vi "Init_Horizontal_ROI.vi"(8 "error in (no error)":errorcluster, 10 "input cluster":T1={"Mode"=enum."ROI", "Manual LUT"={"Minimum"=0.0, "Maximum"=0.0}, "BCG Values"={"Brightness"=128.0, "Contrast"=45.0, "Gamma"=1.0}, "ImageProcessed"=refnum, "Image "=refnum, "Log?"=FALSE, "Auto?"=FALSE, "ROI"={"Global Rectangle"=[], "Contours"=[]}, "ROI Parameters"={"Count"=0.0, "Size(um)"=0.0}, "Image X"=0, "Image Y"=0, "Horizontal ROI"={"Global Rectangle"=[], "Contours"=[]}, "HROI Pos"=0, "Custom ROI"={"Global Rectangle"=[], "Contours"=[]}, "Intensity Graph"=[]} {"ROI Parameters"."Size(um)" min=0 max=255 step=0.1 format="%.2f"; "ROI Parameters"."Count" min=0 max=255 step=0.1 format="%.2f"}) -> (0 "error out":errorcluster, 2 "output cluster":T1={"Mode"=enum."ROI", "Manual LUT"={"Minimum"=0.0, "Maximum"=0.0}, "BCG Values"={"Brightness"=128.0, "Contrast"=45.0, "Gamma"=1.0}, "ImageProcessed"=refnum, "Image "=refnum, "Log?"=FALSE, "Auto?"=FALSE, "ROI"={"Global Rectangle"=[], "Contours"=[]}, "ROI Parameters"={"Count"=0.0, "Size(um)"=0.0}, "Image X"=0, "Image Y"=0, "Horizontal ROI"={"Global Rectangle"=[], "Contours"=[]}, "HROI Pos"=0, "Custom ROI"={"Global Rectangle"=[], "Contours"=[]}, "Intensity Graph"=[]} {"ROI Parameters"."Size(um)" min=0 max=255 step=0.1 format="%.2f"; "ROI Parameters"."Count" min=0 max=255 step=0.1 format="%.2f"})   [LabVIEW 2023, in "Camera_Controller.lvlib"]
uses:
  Camera_Controller.lvlib
  typedefs/ImageProcessingParameters.ctl
  <vilib>/vision/Image Controls.llb/IMAQ Image.ctl
  <vilib>/vision/NI_Vision_Development_Module.lvlib
  typedefs/typedefs.lvlib
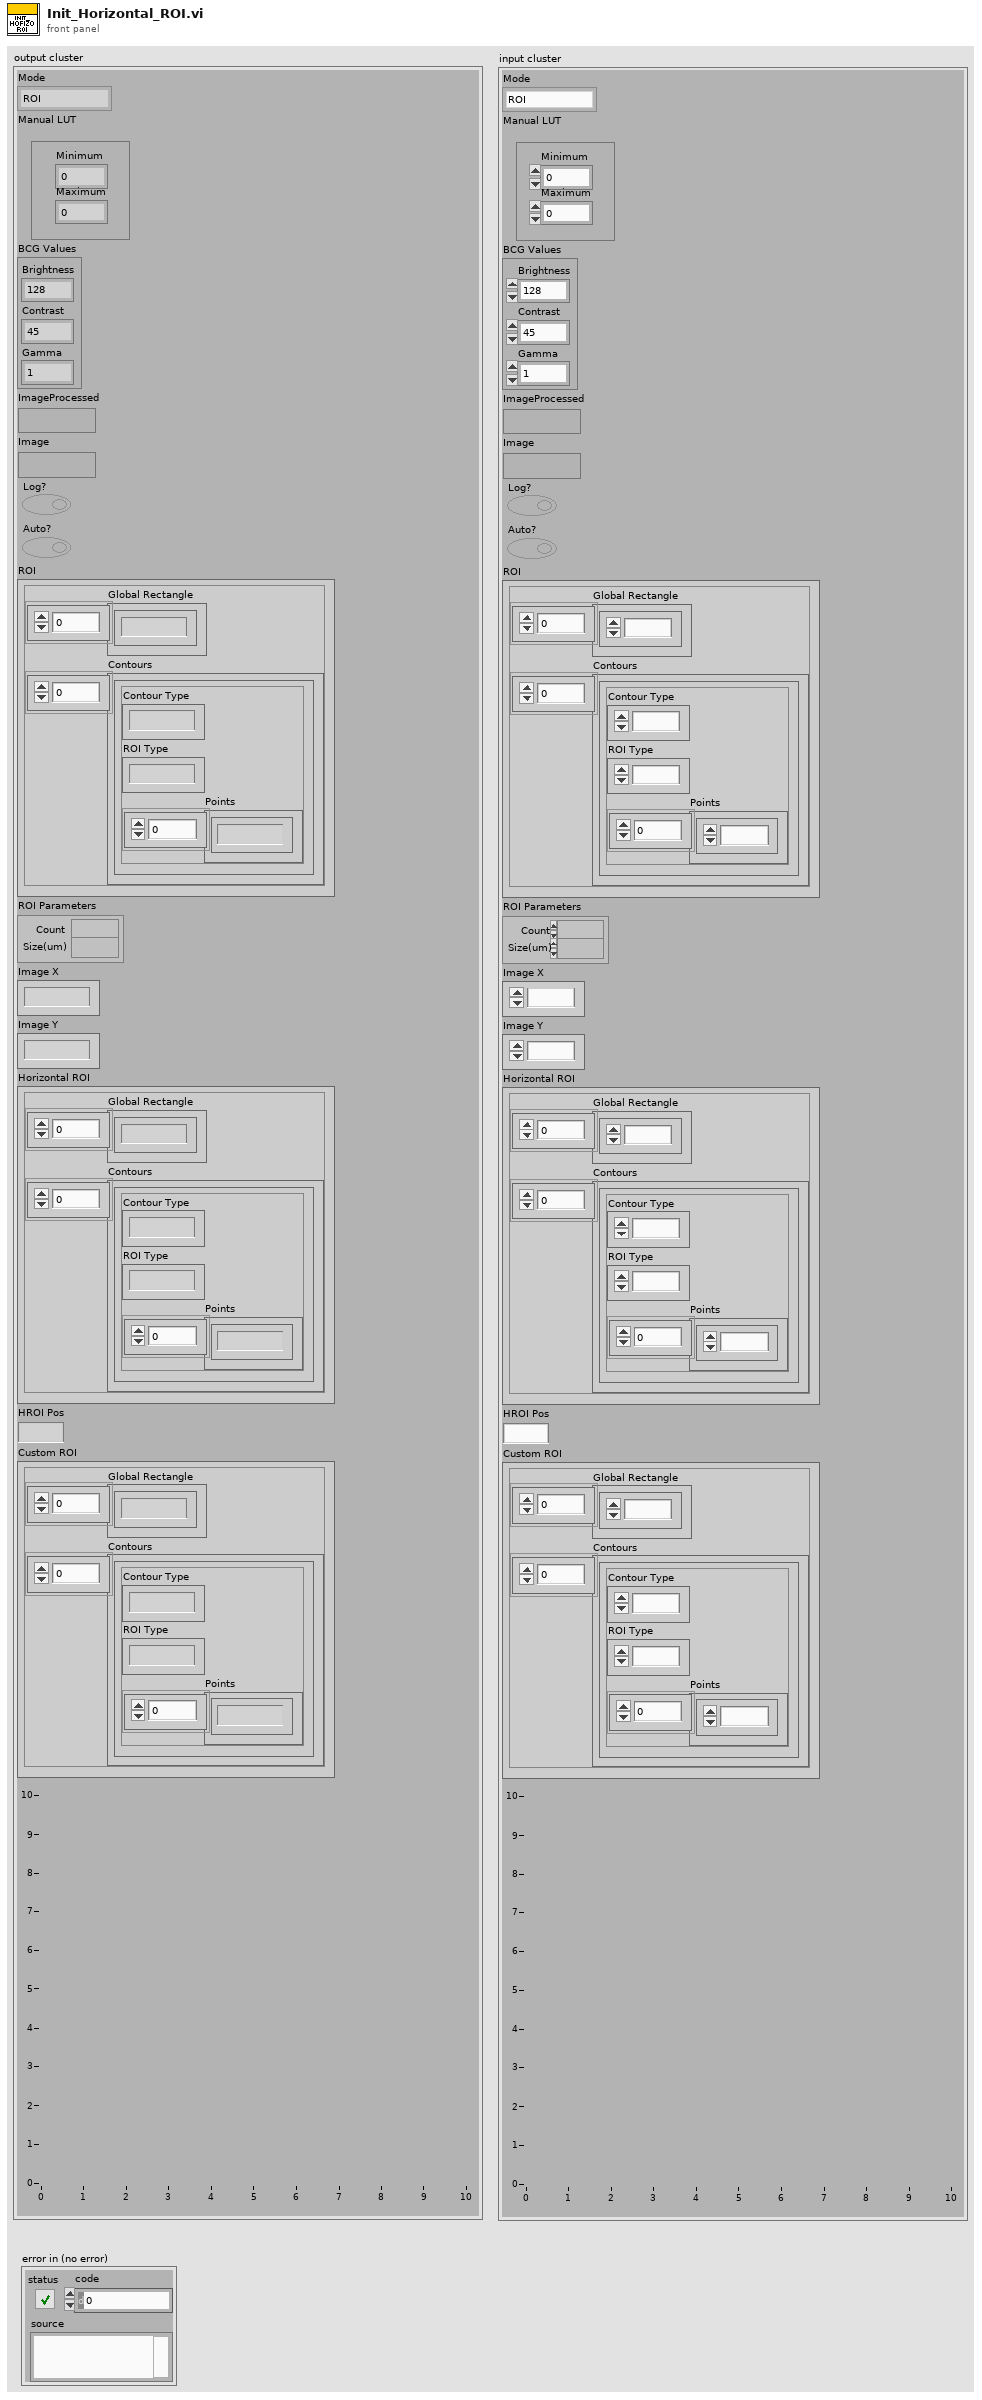
[diagram p1: front panel]
types:
  T1 = typedef "typedefs.lvlib/ImageProcessingParameters.ctl" = cluster{"Mode":enum16{"ROI", "Image"}, "Manual LUT":cluster{"Minimum":dbl, "Maximum":dbl}, "BCG Values":cluster{"Brightness":sgl, "Contrast":sgl, "Gamma":sgl}, "ImageProcessed":T2, "Image ":T2, "Log?":bool, "Auto?":bool, "ROI":cluster{"Global Rectangle":i32[], "Contours":cluster{"Contour Type":u32, "ROI Type":u32, "Points":i32[]}[]}, "ROI Parameters":cluster{"Count":sgl, "Size(um)":sgl}, "Image X":i32, "Image Y":i32, "Horizontal ROI":cluster{"Global Rectangle":i32[], "Contours":cluster{"Contour Type":u32, "ROI Type":u32, "Points":i32[]}[]}, "HROI Pos":u16, "Custom ROI":cluster{"Global Rectangle":i32[], "Contours":cluster{"Contour Type":u32, "ROI Type":u32, "Points":i32[]}[]}, "Intensity Graph":u8[][]}
  T2 = typedef "IMAQ Image.ctl" = refnum<image>
  T3 = cluster{"x1Left":i32, "y1Top":i32, "x2Right":i32, "y2Bottom":i32}
  T4 = typedef "ROI Descriptor" = cluster{"Global Rectangle":i32[], "Contours":cluster{"ID":enum32{"External", "Internal"}, "Type":u32, "Coordinates":i32[]}[]}
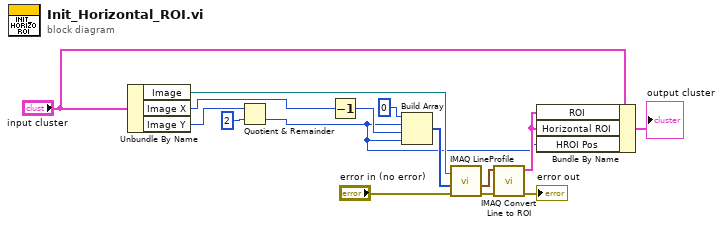
[diagram p0: block diagram]
diagram:
  n1 = Unbundle By Name("input cluster") -> ("Image"=w10:T2, "Image X"=w6:i32, "Image Y"=w3:i32)
  n2 = Quotient & Remainder(x=w3, y=2) -> (floor(x/y)=w1:i32)  [unwired: 1 out]
  n3 = Decrement(x=w6) -> (x-1=w5:i32)
  n4 = Build Array(u16 0 ("element"), w1, w5, w1) -> (w7:i32[])
  n5 = call "IMAQ LineProfile"("error in (no error)"="error in (no error)", "Line Coordinates"=w7, "Image"=w10) -> ("Global Rectangle"=w11:T3, "error out"=w15:errorcluster)  [unwired: 2 in, 2 out]
  n6 = call "IMAQ Convert Line to ROI"("error in (no error)"=w15, "Line"=w11) -> ("error out"=→"error out":errorcluster, "ROI Descriptor"=w4:T4)  [unwired: 7 in]
  n7 = Bundle By Name(cluster="input cluster", "ROI"=w4, "Horizontal ROI"=w4, "HROI Pos"=w1) -> (→"output cluster":T1)
